vi "CC Script Next Dither.vi"(8 "error in (no error)":errorcluster, 10 "object":T2={"Object"={"Name"=""}, "Sidereal Rate"={"dRA"=0.0, "dDEC"=0.0}, "RA and DEC"={"RA"=0.0, "DEC"=0.0}, "Proper Motion"={"muRA"=0.0, "muDEC"=0.0, "Epoch"=0.0}, "Offsets"={"xi"=0.0, "eta"=0.0, "Offset Type"=enum."SIMPLE"}, "Equinox"={"Equinox Year"=2000, "Equinox Prefix"="J"}, "Parallax"={"Parallax"=0.0, "rv kps"=0.0}, "Rotator"={"Frame"=enum."Target", "PA"=0.0}, "Frame"=enum."FK5", "Frac Rate"=1.0, "Wavelength"=0.5}, 11 "Dither":T10) -> (0 "error out":errorcluster, 1 "Dither?":bool, 2 "Offsets":T1, 3 "Dither out":T10, 4 "Message":string)   [LabVIEW 2024]
uses:
  typedefs/CC cluster Dithering.ctl
  typedefs/CC cluster Random Dithering.ctl
  typedefs/CC Dithering.ctl
  typedefs/CC cluster Offset Dithering.ctl
  typedefs/CC Dithering Offsets.ctl
  typedefs/CC cluster Object.ctl
  typedefs/CC cluster sidereal rate.ctl
  typedefs/CC cluster RA and DEC.ctl
  typedefs/cc cluster muRA muDEC.ctl
  Telescope/CC cluster Telescope Offsets.ctl
  Telescope/Telescope cluster Equinox.ctl
  Telescope/Telescope cluster Parallax.ctl
  Telescope/Telescope cluster Rotator.ctl
  Telescope/Telesope ring Frame.ctl
  Telescope/LDT Telescope/LDT Telescope.lvclass
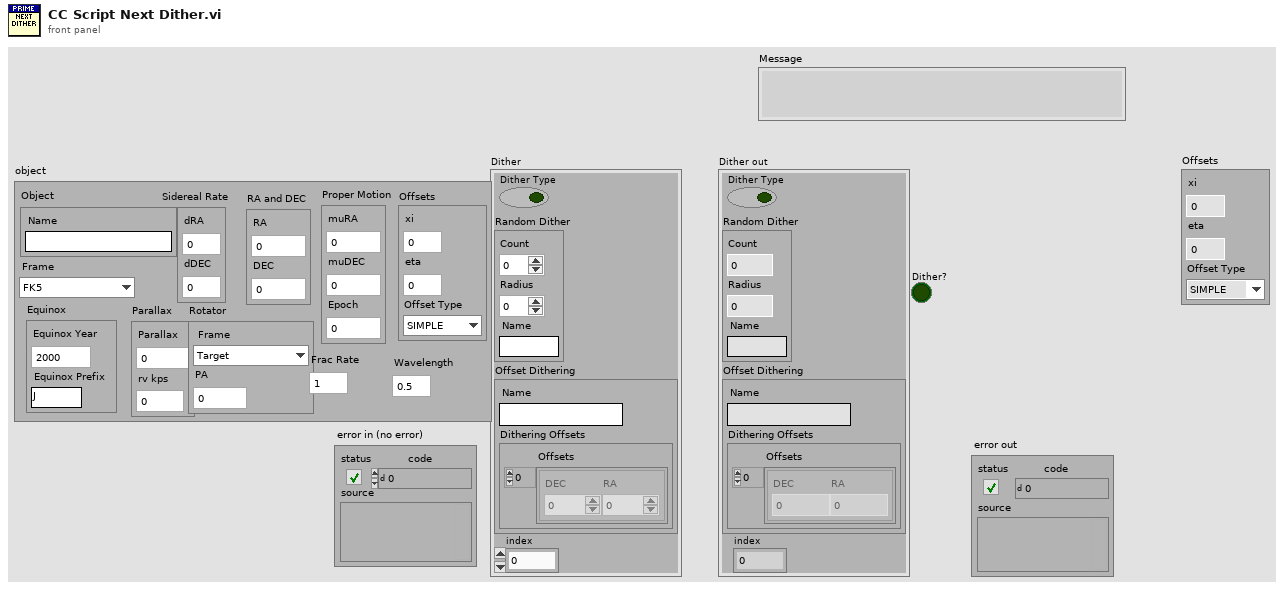
[diagram p1: front panel]
types:
  T1 = typedef "CC cluster Telescope Offsets.ctl" = cluster{"xi":dbl, "eta":dbl, "Offset Type":enum16{"SIMPLE", "TPLANE", "PA"}}
  T2 = typedef "CC cluster Object.ctl" = cluster{"Object":cluster{"Name":string}, "Sidereal Rate":T3, "RA and DEC":T4, "Proper Motion":T5, "Offsets":T1, "Equinox":T6, "Parallax":T7, "Rotator":T8, "Frame":T9, "Frac Rate":dbl, "Wavelength":dbl}
  T3 = typedef "CC cluster sidereal rate.ctl" = cluster{"dRA":dbl, "dDEC":dbl}
  T4 = typedef "CC cluster RA and DEC.ctl" = cluster{"RA":dbl, "DEC":dbl}
  T5 = typedef "cc cluster muRA muDEC.ctl" = cluster{"muRA":dbl, "muDEC":dbl, "Epoch":dbl}
  T6 = typedef "Telescope cluster Equinox.ctl" = cluster{"Equinox Year":i32, "Equinox Prefix":string}
  T7 = typedef "Telescope cluster Parallax.ctl" = cluster{"Parallax":dbl, "rv kps":dbl}
  T8 = typedef "Telescope cluster Rotator.ctl" = cluster{"Frame":enum16{"Target", "Fixed"}, "PA":dbl}
  T9 = typedef "Telesope ring Frame.ctl" = enum16{"FK4", "FK5", "APPT", "GAPPT", "AZEL"}
  T10 = typedef "CC cluster Dithering.ctl" = cluster{"Dither Type":bool, "Random Dither":T11, "Offset Dithering":T12, "index":i32}
  T11 = typedef "CC cluster Random Dithering.ctl" = cluster{"Count":i32, "Radius":dbl, "Name":string}
  T12 = typedef "CC Dithering.ctl" = cluster{"Name":string, "Dithering Offsets":T13}
  T13 = typedef "CC cluster Offset Dithering.ctl" = cluster{"Offsets":T14[]}
  T14 = typedef "CC Dithering Offsets.ctl" = cluster{"DEC":dbl, "RA":dbl}
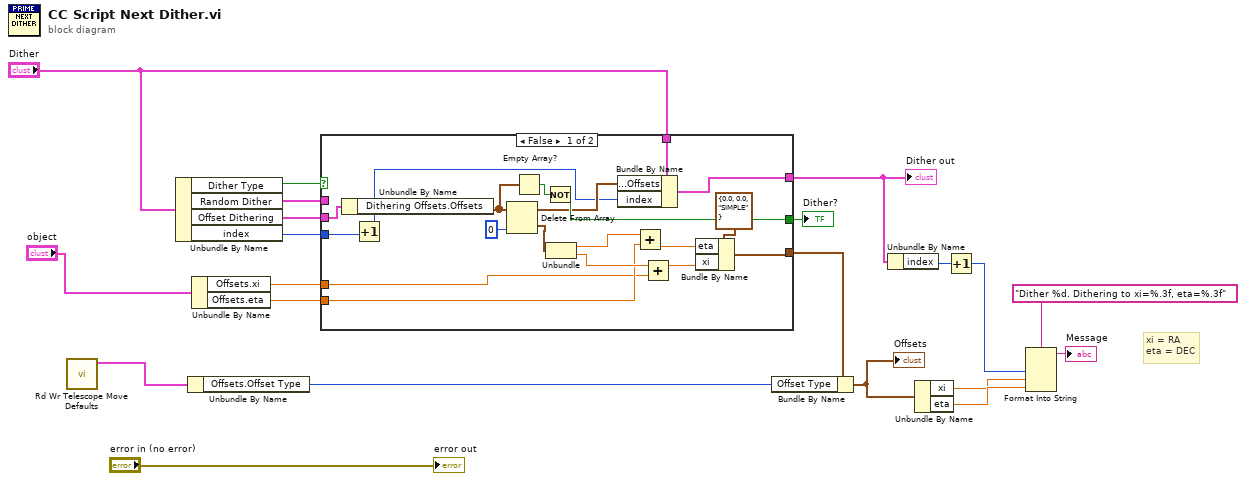
[diagram p0: block diagram]
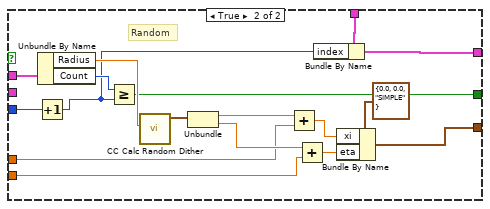
[diagram p2: hidden frame]
diagram:
  # "xi = RA\neta = DEC"
  n1 = call "Rd Wr Telescope Move Defaults.vi"() -> ("Move Position"=w2:T2)  [unwired: 10 in, 1 out]
  n2 = Unbundle By Name("Dither") -> ("Dither Type"=w20:bool, "Random Dither"=w19:T11, "Offset Dithering"=w17:T12, "index"=w18:i32)
  n3 = Unbundle By Name(w2) -> ("Offsets.Offset Type"=w1:enum16{"SIMPLE", "TPLANE", "PA"})
  n4 = Unbundle By Name("object") -> ("Offsets.xi"=w6:dbl, "Offsets.eta"=w5:dbl)
  n5 = case shown="False" w20 {
    tunnel: w19 -> [_ w57]
    tunnel: w18 -> [w32 w56]
    tunnel: w17 -> [w40 _]
    tunnel: [w36 w53] -> w14
    tunnel: [w28 w46] -> w4
    tunnel: "Dither" -> [w35 w51]
    tunnel: [w33 w50] -> w10
    tunnel: w6 -> [w22 w41]
    tunnel: w5 -> [w23 w43]
    frame False {
      n6 = Unbundle By Name(w40) -> ("Dithering Offsets.Offsets"=w38:T14[])
      n7 = Increment(x=w32) -> (x+1=w31:i32)
      n8 = Delete From Array(array=w38, index=0) -> (deleted portion=w27:T14, array with subset deleted=w34:T14[])  [unwired: 1 in]
      n9 = Empty Array?(array=w38) -> (empty?=w37:bool)
      n10 = Not(x=w37) -> (.not. x?=w36:bool)
      n11 = Unbundle(w27) -> ("DEC"=w30:dbl, "RA"=w29:dbl)
      n12 = Bundle By Name(cluster=w35, "Offset Dithering.Dithering Offsets.Offsets"=w34, "index"=w31) -> (w33:T10)
      n13 = Add(x=w30, y=w23) -> (x+y=w25:dbl)
      n14 = Add(x=w29, y=w22) -> (x+y=w24:dbl)
      n15 = Bundle By Name(cluster=T1 {"xi"=0.0, "eta"=0.0, "Offset Type"=enum."SIMPLE"} ("Offsets"), "eta"=w25, "xi"=w24) -> (w28:T1)
    }
    frame True {
      # "Random"
      n16 = Increment(x=w56) -> (x+1=w52:i32)
      n17 = Unbundle By Name(w57) -> ("Radius"=w54:dbl, "Count"=w55:i32)
      n18 = Greater Or Equal?(x=w55, y=w52) -> (x >= y?=w53:bool)
      n19 = call "CC Calc Random Dither.vi"("Radius (arcsec)"=w54) -> ("Dither RA and DEC"=w49:T4)  [unwired: 9 in, 1 out]
      n20 = Unbundle(w49) -> ("RA"=w48:dbl, "DEC"=w47:dbl)
      n21 = Add(x=w48, y=w41) -> (x+y=w42:dbl)
      n22 = Add(x=w47, y=w43) -> (x+y=w44:dbl)
      n23 = Bundle By Name(cluster=w51, "index"=w52) -> (w50:T10)
      n24 = Bundle By Name(cluster=T1 {"xi"=0.0, "eta"=0.0, "Offset Type"=enum."SIMPLE"} ("Offsets"), "xi"=w42, "eta"=w44) -> (w46:T1)
    }
  }
  "Dither out" <- w10
  "Dither?" <- w14
  n25 = Bundle By Name(cluster=w4, "Offset Type"=w1) -> (w3:T1)
  "Offsets" <- w3
  n26 = Unbundle By Name(w10) -> ("index"=w8:i32)
  n27 = Unbundle By Name(w3) -> ("xi"=w9:dbl, "eta"=w12:dbl)
  n28 = Increment(x=w8) -> (x+1=w7:i32)
  n29 = Format Into String(format string="Dither %d. Dithering to xi=%.3f, eta=%.3f", w7, w9, w12) -> (resulting string=→"Message":string)  [unwired: 2 in, 1 out]
  "error out" <- "error in (no error)"
